vi "E Read cells.vi"(0 "Excel._Worksheet":refnum<k7>, 5 "Cells/表格位置":string, 11 "error in (no error)":errorcluster) -> (4 "Excel._Worksheet":refnum<k7>, 6 "Excel.Range":refnum<k7>, 8 "Array data/二维数据":string[][](array[string]), 15 "error out":errorcluster)   [LabVIEW 2014]
doc: "从指定的单元格里读取一个二维数组。"
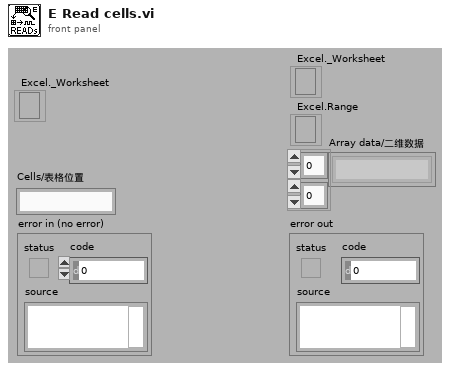
[diagram p1: front panel]
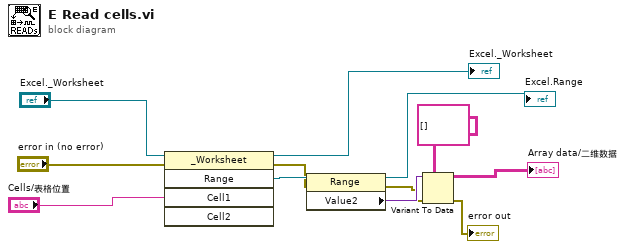
[diagram p0: block diagram]
diagram:
  n1 = invoke class="_Worksheet" method="Range"(reference="Excel._Worksheet", error in="error in (no error)", "Cell1"="Cells/表格位置") -> (reference out=→"Excel._Worksheet":refnum<k7>, error out=w8:errorcluster, "Range"=w9:refnum<k7>)  [unwired: 2 in, 2 out]
  n2 = property class="Range"(reference=w9, error in=w8) -> (reference out=→"Excel.Range":refnum<k7>, error out=w6:errorcluster, "Value2"=w7:variant)
  n3 = Variant To Data(error in=w6, type=string[][] [], Variant=w7) -> (data=→"Array data/二维数据":string[][], error out=→"error out":errorcluster)
